vi "Read Interface.lvclass.vi"(8 "error in (no error)":errorcluster, 11 "JSON reader in":refnum<class "JSON reader.lvclass">) -> (0 "error out":errorcluster, 2 "Interface.lvclass":refnum<class "Interface.lvclass">, 3 "JSON reader out":refnum<class "JSON reader.lvclass">)   [LabVIEW 2018, in "JSON reader.lvclass"]
uses:
  JSON reader.lvclass
  Interface/Interface.lvclass
  JSON reader.lvclass/JSON reader.ctl
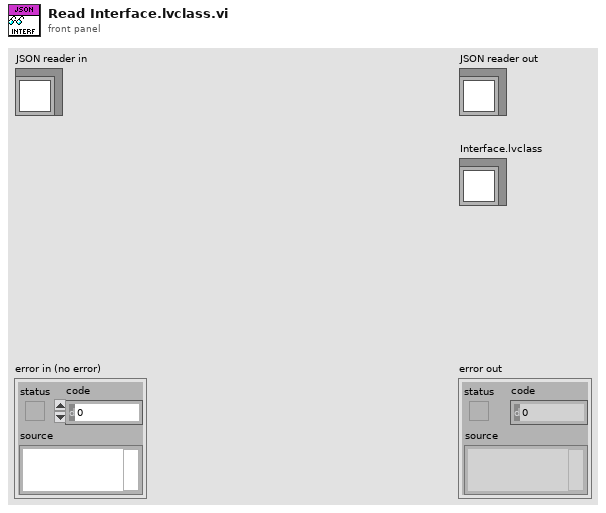
[diagram p1: front panel]
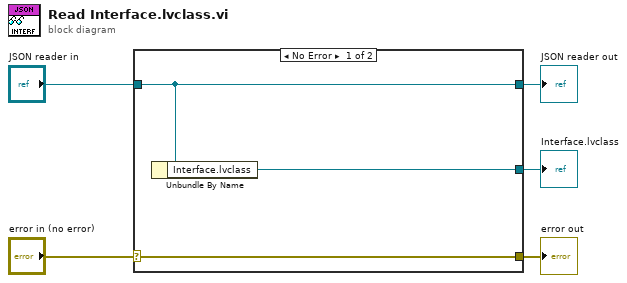
[diagram p0: block diagram]
diagram:
  n1 = case shown="No Error" "error in (no error)" {
    selector: "error in (no error)" -> [w8 w9]
    tunnel: [w8 w9] -> w4
    tunnel: [w7 w10] -> w2
    tunnel: "JSON reader in" -> [w7 w10]
    tunnel: [w6 _] -> w1
    frame No Error {
      n2 = Unbundle By Name(w7) -> ("Interface.lvclass"=w6:refnum<class "Interface.lvclass">)
    }
    frame Error {
    }
  }
  "error out" <- w4
  "JSON reader out" <- w2
  "Interface.lvclass" <- w1
